vi "Clean Up Actor.vi"(8 "error in (no error)":errorcluster, 11 "Replay in":refnum<class "Replay.lvclass">) -> (0 "error out":errorcluster, 3 "Replay out":refnum<class "Replay.lvclass">)   [LabVIEW 2016, in "CLD Exam - ATM.lvlib" / "Replay.lvclass"]
uses:
  Replay.lvclass
  D:/Repos/Stream/software/Mediator/Classes/Mediated Actor/Mediated Actor.lvclass
  Mediator/Classes/Message Broker Interface/Message Broker Interface.lvclass
  Mediator/Classes/Mediated Synchronous Actor/Mediated Synchronous Actor.lvclass
  Mediator/Classes/Mediated Actor/Mediated Actor.lvclass
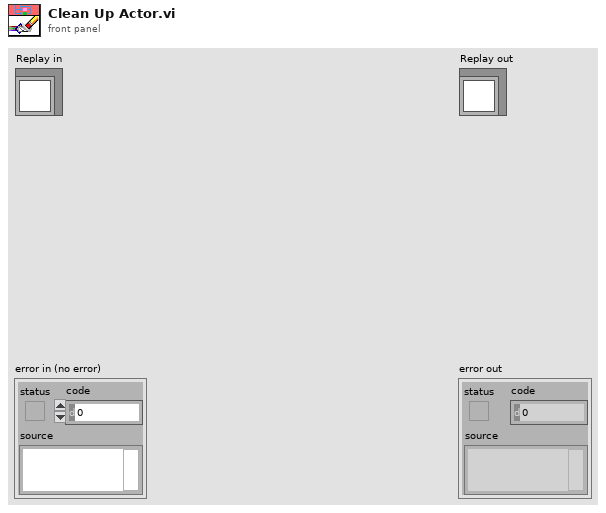
[diagram p1: front panel]
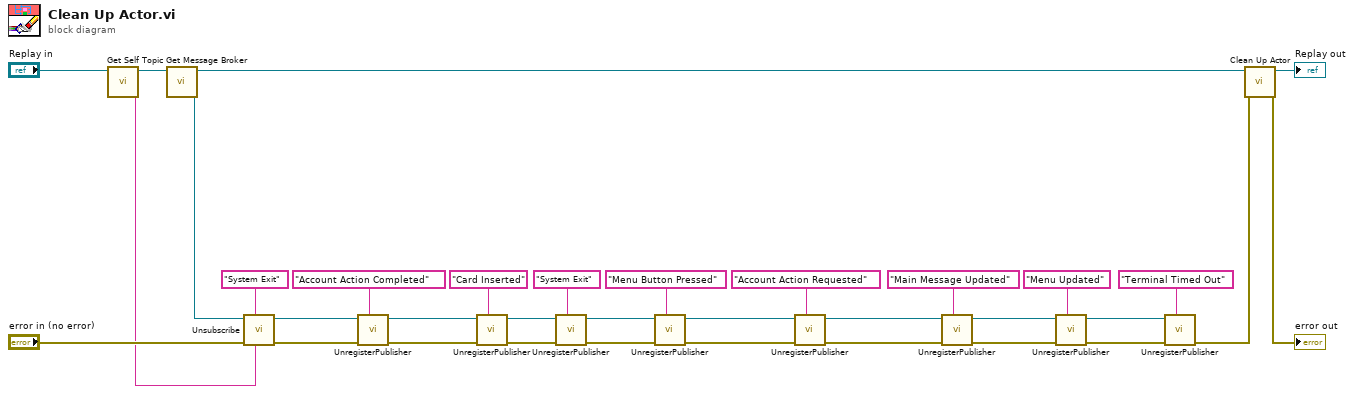
[diagram p0: block diagram]
diagram:
  n1 = call "Get Self Topic.vi"("Mediated Actor in"="Replay in") -> ("Topic.Self"=w25:string, "Mediated Actor out"=w32:refnum<class "Replay.lvclass">)  [unwired: 9 in]
  n2 = call "Get Message Broker.vi"("Mediated Actor in"=w32) -> ("Message Broker"=w26:refnum<class "Message Broker Interface.lvclass">, "Mediated Actor out"=w30:refnum<class "Replay.lvclass">)  [unwired: 9 in]
  n3 = call-dynamic "Unsubscribe.vi"("Subscriber Name"=w25, "Topic Name"="System Exit", "error in (no error)"="error in (no error)", "Message Broker Interface in"=w26) -> ("error out"=w24:errorcluster, "Message Broker Interface out"=w23:refnum<class "Message Broker Interface.lvclass">)  [unwired: 6 in]
  n4 = call-dynamic "UnregisterPublisher.vi"("Topic Name"="Account Action Completed", "error in (no error)"=w24, "Message Broker Interface in"=w23) -> ("error out"=w20:errorcluster, "Message Broker Interface out"=w21:refnum<class "Message Broker Interface.lvclass">)  [unwired: 7 in]
  n5 = call-dynamic "UnregisterPublisher.vi"("Topic Name"="Card Inserted", "error in (no error)"=w20, "Message Broker Interface in"=w21) -> ("error out"=w17:errorcluster, "Message Broker Interface out"=w18:refnum<class "Message Broker Interface.lvclass">)  [unwired: 7 in]
  n6 = call-dynamic "UnregisterPublisher.vi"("Topic Name"="System Exit", "error in (no error)"=w17, "Message Broker Interface in"=w18) -> ("error out"=w14:errorcluster, "Message Broker Interface out"=w15:refnum<class "Message Broker Interface.lvclass">)  [unwired: 7 in]
  n7 = call-dynamic "UnregisterPublisher.vi"("Topic Name"="Menu Button Pressed", "error in (no error)"=w14, "Message Broker Interface in"=w15) -> ("error out"=w11:errorcluster, "Message Broker Interface out"=w12:refnum<class "Message Broker Interface.lvclass">)  [unwired: 7 in]
  n8 = call-dynamic "UnregisterPublisher.vi"("Topic Name"="Account Action Requested", "error in (no error)"=w11, "Message Broker Interface in"=w12) -> ("error out"=w8:errorcluster, "Message Broker Interface out"=w9:refnum<class "Message Broker Interface.lvclass">)  [unwired: 7 in]
  n9 = call-dynamic "UnregisterPublisher.vi"("Topic Name"="Main Message Updated", "error in (no error)"=w8, "Message Broker Interface in"=w9) -> ("error out"=w2:errorcluster, "Message Broker Interface out"=w3:refnum<class "Message Broker Interface.lvclass">)  [unwired: 7 in]
  n10 = call-dynamic "UnregisterPublisher.vi"("Topic Name"="Menu Updated", "error in (no error)"=w2, "Message Broker Interface in"=w3) -> ("error out"=w7:errorcluster, "Message Broker Interface out"=w6:refnum<class "Message Broker Interface.lvclass">)  [unwired: 7 in]
  n11 = call-dynamic "UnregisterPublisher.vi"("Topic Name"="Terminal Timed Out", "error in (no error)"=w7, "Message Broker Interface in"=w6) -> ("error out"=w1:errorcluster)  [unwired: 7 in, 1 out]
  n12 = call-parent "Clean Up Actor.vi"("error in (no error)"=w1, "Mediated Actor in"=w30) -> ("error out"=→"error out":errorcluster, "Mediated Actor out"=→"Replay out":refnum<class "Replay.lvclass">)  [unwired: 8 in]
